vi "StrDimantle.vi"(11 "StrIn":string) -> (0 "上限值":dbl, 1 "下限值":dbl, 2 "循环次数":i32, 3 "Audio":string)   [LabVIEW 2013]
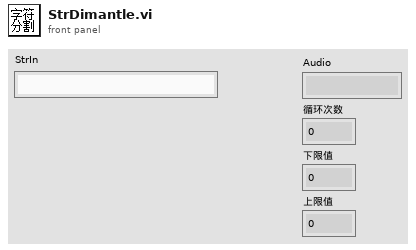
[diagram p1: front panel]
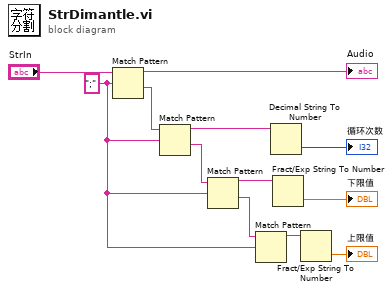
[diagram p0: block diagram]
diagram:
  w7 = ";"
  n1 = Match Pattern(string="StrIn", regular expression=w7) -> (before substring=→"Audio":string, after substring=w10:string)  [unwired: 1 in, 2 out]
  n2 = Match Pattern(string=w10, regular expression=w7) -> (before substring=w6:string, after substring=w9:string)  [unwired: 1 in, 2 out]
  n3 = Match Pattern(string=w9, regular expression=w7) -> (before substring=w4:string, after substring=w8:string)  [unwired: 1 in, 2 out]
  n4 = Match Pattern(string=w8, regular expression=w7) -> (before substring=w2:string)  [unwired: 1 in, 3 out]
  n5 = Decimal String To Number(string=w6) -> (number=→"循环次数":i32)  [unwired: 2 in, 1 out]
  n6 = Fract/Exp String To Number(string=w4) -> (number=→"下限值":dbl)  [unwired: 3 in, 1 out]
  n7 = Fract/Exp String To Number(string=w2) -> (number=→"上限值":dbl)  [unwired: 3 in, 1 out]
